vi "TGA.vi"(0 "System no.":i32=1 min=1 max=4 step=1, 2 "Trajectory ID":i32[](array[numeric]), 3 "Trajectory values":dbl[](array[numeric]) format="%.6f", 4 "No.of digits":i16=4, 5 "error in":errorcluster) -> (19 "error out":errorcluster)   [LabVIEW 2020]
doc: "Append values to trajectories. For further details, see Trajectories for Motion Paths in the controller user manual.\n\nC-867, C-884:"
panel:
  # "Append values to trajectories."
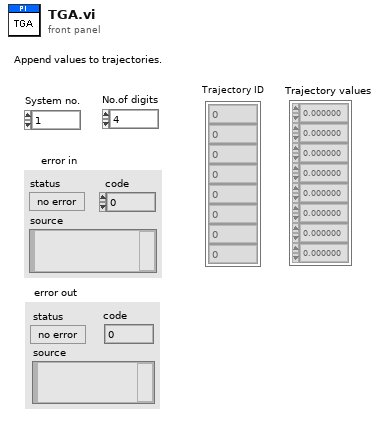
[diagram p1: front panel]
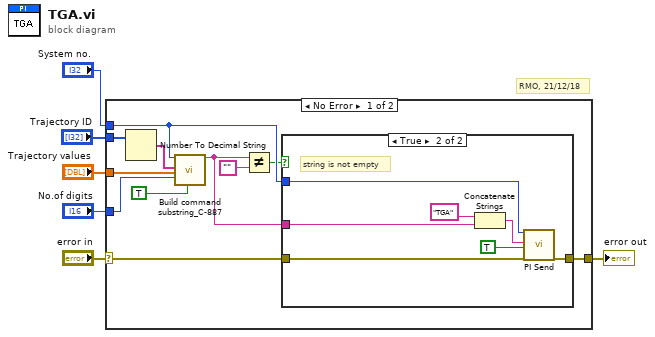
[diagram p0: block diagram]
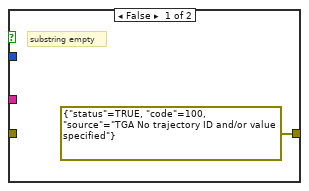
[diagram p2: hidden frame]
diagram:
  # "RMO, 21/12/18"
  n1 = case shown="No Error" "error in" {
    selector: "error in" -> [w7 w26]
    tunnel: [w17 w26] -> w6
    tunnel: "Trajectory values" -> [w14 _]
    tunnel: "No.of digits" -> [w13 _]
    tunnel: "System no." -> [w12 _]
    tunnel: "Trajectory ID" -> [w8 _]
    frame No Error {
      n2 = Number To Decimal String(number=w8) -> (decimal integer string=w9:string[])  [unwired: 1 out]
      n3 = call "Build command substring_C-887.vi"("System no."=w12, "Affected axes"=w9, "Parameters"=w14, "No. of digits"=w13, "With space?"=TRUE) -> ("Command substring"=w15:string)  [unwired: 2 in, 12 out]
      n4 = Not Equal?(x=w15, y="") -> (x != y?=w11:bool)
      n5 = case shown="True" w11 {
        tunnel: w15 -> [_ w24]
        tunnel: [errorcluster {"status"=TRUE, "code"=100, "source"="TGA No trajectory ID and/or value specified"} ("error out") w20] -> w17
        tunnel: w7 -> [_ w21]
        tunnel: w12 -> [_ w19]
        frame False {
          # "substring empty"
        }
        frame True {
          # "string is not empty"
          n6 = Concatenate Strings("TGA", w24) -> (w22:string)
          n7 = call "PI Send.vi"("System no."=w19, "String to send"=w22, "Attach termination char.?"=TRUE ("Attach Linefeed?"), "error in"=w21) -> ("error out"=w20:errorcluster)  [unwired: 2 in, 13 out]
        }
      }
    }
    frame Error {
    }
  }
  "error out" <- w6
